vi "ep_Interpolate Load and Efficiency.vi"(5 "algorithm":T1, 7 "index":i32, 9 "total input active power [W]":dbl, 10 "full load [W]":dbl, 11 "efficiency values [%]":dbl[](array[numeric])) -> (1 "efficiency [%]":dbl, 3 "load [W]":dbl)   [LabVIEW 2014, in "NI_EP_Motor Monitoring.lvlib"]
uses:
  <vilib>/addons/Electrical Power/Motor Monitoring/NI_EP_Motor Monitoring.lvlib
  <vilib>/addons/Electrical Power/Motor Monitoring/subVIs/ep_Input Power Algorithm.ctl
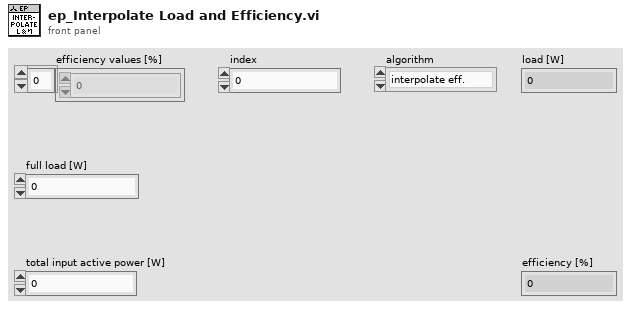
[diagram p1: front panel]
types:
  T1 = typedef "NI_EP_Motor Monitoring.lvlib/ep_Input Power Algorithm.ctl" = enum16{"interpolate eff.", "use min eff.", "use default eff."}
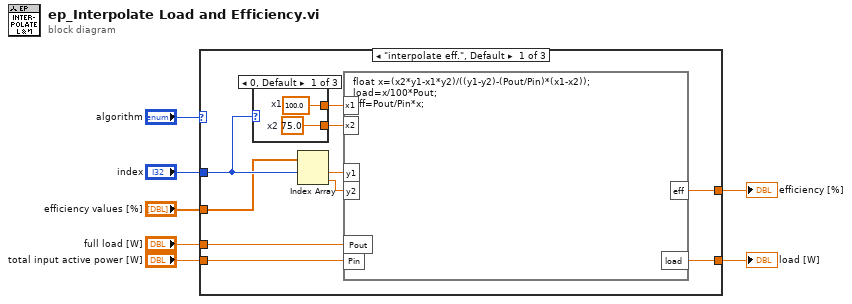
[diagram p0: block diagram]
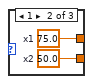
[diagram p2: hidden frame]
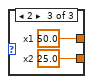
[diagram p3: hidden frame]
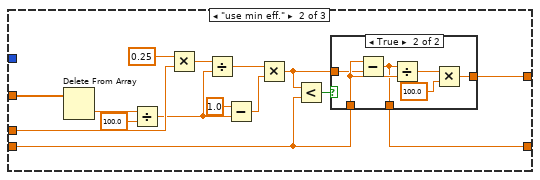
[diagram p4: hidden frame]
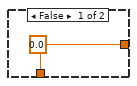
[diagram p5: hidden frame]
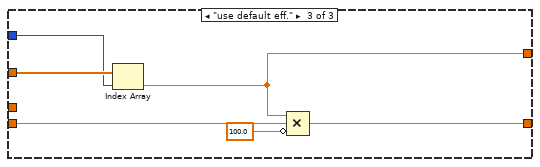
[diagram p6: hidden frame]
diagram:
  n1 = case shown="\"interpolate eff.\", Default" "algorithm" {
    tunnel: "efficiency values [%]" -> [w8 w25 w48]
    tunnel: [w9 w27 w47] -> w7
    tunnel: "total input active power [W]" -> [w12 w28 w50]
    tunnel: [w10 w26 w51] -> w5
    tunnel: "index" -> [w17 _ w46]
    tunnel: "full load [W]" -> [w11 w35 _]
    frame "interpolate eff.", Default {
      n2 = case shown="0, Default" w17 {
        tunnel: [w19 w21 w23] -> w16
        tunnel: [w18 w20 w22] -> w15
        frame 0, Default {
          w18 = 75.0  # x2
          w19 = 100.0  # x1
        }
        frame 1 {
          w20 = 50.0  # x2
          w21 = 75.0  # x1
        }
        frame 2 {
          w22 = 25.0  # x2
          w23 = 50.0  # x1
        }
      }
      n3 = Index Array(array=w8, index #1=w17) -> (element #1=w14:dbl, element #2=w13:dbl)  [unwired: 1 in]
      n4 = formula code="float x=(x2*y1-x1*y2)/((y1-y2)-(Pout/Pin)*(x1-x2));\nload=x/100*Pout;\neff=Pout/Pin*x;"("x1"=w16, "x2"=w15, "y1"=w14, "y2"=w13, "Pin"=w12, "Pout"=w11) -> ("eff"=w9:dbl, "load"=w10:dbl)
    }
    frame "use min eff." {
      n5 = Delete From Array(array=w25) -> (deleted portion=w38:dbl)  [unwired: 2 in, 1 out]
      n6 = Divide(x=w38, y=100.0 ("value")) -> (x/y=w33:dbl)
      n7 = Multiply(x=0.25, y=w35) -> (x*y=w36:dbl)
      n8 = Divide(x=w36, y=w33) -> (x/y=w34:dbl)
      n9 = Subtract(x=1.0 ("value"), y=w33) -> (x-y=w31:dbl)
      n10 = Multiply(x=w34, y=w31) -> (x*y=w30:dbl)
      n11 = Less?(x=w30, y=w28) -> (x < y?=w29:bool)
      n12 = case shown="True" w29 {
        tunnel: [w39 w42] -> w27
        tunnel: w30 -> [_ w41]
        tunnel: w28 -> [_ w43]
        tunnel: [w39 w40] -> w26
        frame False {
          w39 = 0.0
        }
        frame True {
          n13 = Subtract(x=w43, y=w41) -> (x-y=w40:dbl)
          n14 = Divide(x=w40, y=w43) -> (x/y=w44:dbl)
          n15 = Multiply(x=w44, y=100.0 ("value")) -> (x*y=w42:dbl)
        }
      }
    }
    frame "use default eff." {
      n16 = Index Array(array=w48, index=w46) -> (element=w47:dbl)
      n17 = Compound Arithmetic op=MULTIPLY(w47, w50, invert 100.0 ("value")) -> (w51:dbl)
    }
  }
  "load [W]" <- w5
  "efficiency [%]" <- w7
